vi "Pane size change.vi"(8 "error in (no error)":errorcluster, 10 "Control refs":variant) -> (0 "error out":errorcluster)   [LabVIEW 2018, in "Monitored Actor.lvlib" / "Actor Monitor.lvclass"]
doc: "Repositions everything in the UI after the panel has been resized. Use the control names to lookup the references in the variant\n\nCopyright: MGI\nAuthored by: Derek Trepanier"
uses:
  Actor Monitor.lvclass
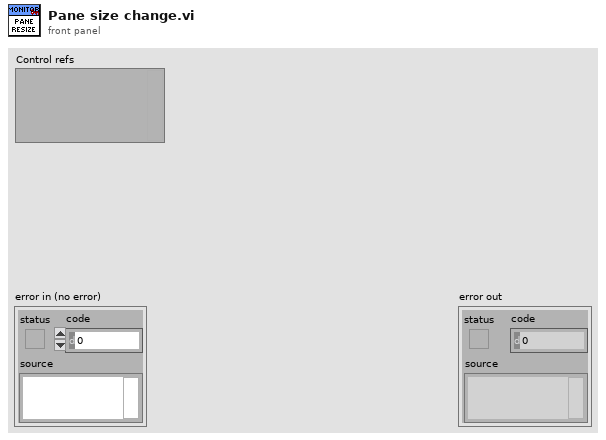
[diagram p1: front panel]
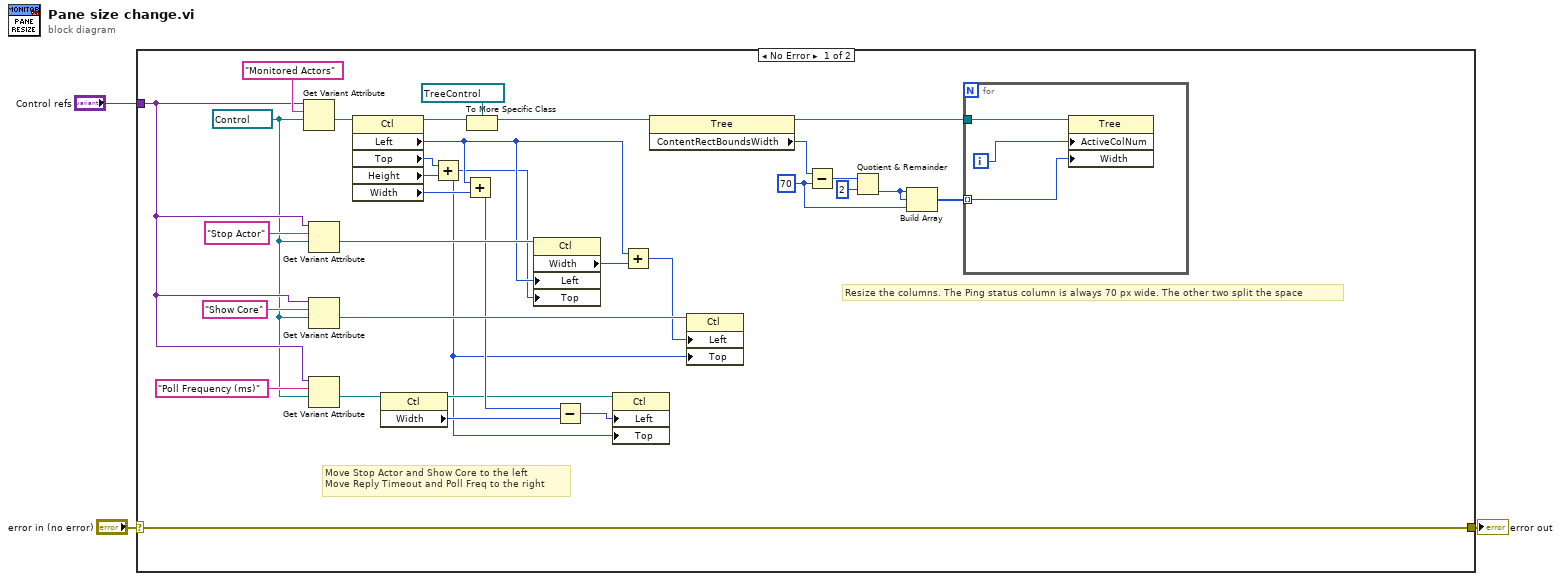
[diagram p0: block diagram]
diagram:
  n1 = case shown="No Error" "error in (no error)" {
    selector: "error in (no error)" -> [w35 w39]
    tunnel: [w35 w39] -> w2
    tunnel: "Control refs" -> [w20 _]
    frame No Error {
      w5 = 70 ("y")
      w18 = refnum<vi> refnum ("reference out")
      # "Resize the columns. The Ping status column is always 70 px wide. The other two split the space"
      # "Move Stop Actor and Show Core to the left\nMove Reply Timeout and Poll Freq to the right"
      n2 = Get Variant Attribute(Variant=w20, name="Monitored Actors", default value (empty Variant)=w18) -> (value=w33:refnum<vi>)  [unwired: 1 in, 3 out]
      n3 = Get Variant Attribute(Variant=w20, name="Stop Actor", default value (empty Variant)=w18) -> (value=w28:refnum<vi>)  [unwired: 1 in, 3 out]
      n4 = Get Variant Attribute(Variant=w20, name="Show Core", default value (empty Variant)=w18) -> (value=w24:refnum<vi>)  [unwired: 1 in, 3 out]
      n5 = Get Variant Attribute(Variant=w20, name="Poll Frequency (ms)", default value (empty Variant)=w18) -> (value=w21:refnum<vi>)  [unwired: 1 in, 3 out]
      n6 = property class="Ctl"(reference=w33) -> (reference out=w13:refnum<vi>, "Left"=w26:i32, "Top"=w32:i32, "Height"=w31:u32, "Width"=w30:u32)  [unwired: 1 in, 1 out]
      n7 = property class="Ctl"(reference=w21) -> (reference out=w16:refnum<vi>, "Width"=w17:u32)  [unwired: 1 in, 1 out]
      n8 = Add(x=w32, y=w31) -> (x+y=w14:u32)
      n9 = Add(x=w26, y=w30) -> (x+y=w22:u32)
      n10 = To More Specific Class(target class=refnum<vi> refnum ("reference out"), reference=w13) -> (specific class reference=w11:refnum<vi>)  [unwired: 1 in, 1 out]
      n11 = property class="Ctl"(reference=w28, "Left"=w26, "Top"=w14) -> ("Width"=w27:u32)  [unwired: 1 in, 2 out]
      n12 = Subtract(x=w22, y=w17) -> (x-y=w15:u32)
      n13 = property class="Ctl"(reference=w16, "Left"=w15, "Top"=w14) -> ()  [unwired: 1 in, 2 out]
      n14 = Add(x=w26, y=w27) -> (x+y=w23:u32)
      n15 = property class="Tree"(reference=w11) -> (reference out=w10:refnum<vi>, "ContentRectBoundsWidth"=w9:i32)  [unwired: 1 in, 1 out]
      n16 = property class="Ctl"(reference=w24, "Left"=w23, "Top"=w14) -> ()  [unwired: 1 in, 2 out]
      n17 = Subtract(x=w9, y=w5) -> (x-y=w8:i32)
      n18 = Quotient & Remainder(x=w8, y=2) -> (floor(x/y)=w6:i32)  [unwired: 1 out]
      n19 = Build Array(w6, w6, w5) -> (w4:i32[])
      n20 = for {
        tunnel: w10 -> [w38]
        tunnel: w4 -> [w37] mode=indexing
        i -> [w36]
        n21 = property class="Tree"(reference=w38, "ActiveColNum"=w36, "Width"=w37) -> ()  [unwired: 1 in, 2 out]
      }
    }
    frame Error {
    }
  }
  "error out" <- w2
